vi "instrumentProperties_channel_gainLevels_init.vi"(8 "error in (no error)":errorcluster, 11 "OSAchannel in":refnum<class "OSAchannel.lvclass">) -> (0 "error out":errorcluster, 2 "gain values (relative)":dbl[](array[numeric]), 3 "OSAchannel out":refnum<class "OSAchannel.lvclass">)   [LabVIEW 2010, in "OSAchannel.lvclass"]
uses:
  OSAchannel.lvclass
  _dll/LVLib/FTSLib.lvlib
  OSA20X_misc.lvlib
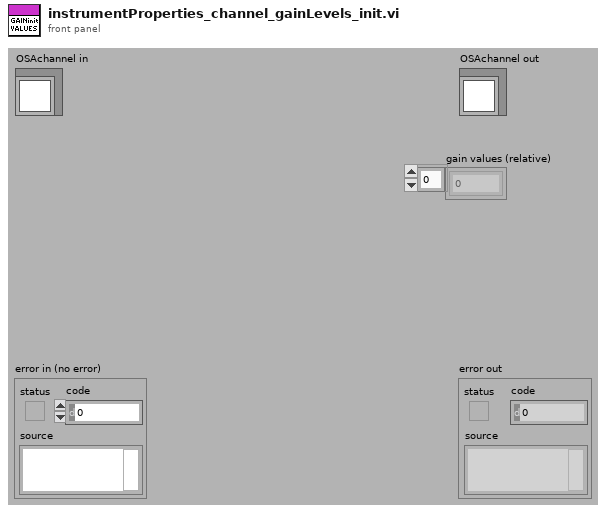
[diagram p1: front panel]
types:
  T1 = typedef "OSA20X_misc.lvlib/amplifier_sort.ctl" = enum16{"amp_unknown", "amp_se_8", "amp_se_12_lg", "amp_se_12", "amp_se_16", "amp_diff_8", "amp_diff_12_lg", "amp_diff_12_ir", "amp_diff_16", "amp_other", "amp_other_2"}
  T2 = typedef "OSA20X_misc.lvlib/detector_sort.ctl" = enum16{"unknown", "Silicon", "Silicon PIN", "Silicon MPPC", "InGaAs", "InGaAs ext low", "InGaAs ext high", "InAs", "InAsSb", "InSb", "MCT", "other", "other2", "other3"}
  T3 = typedef "OSA20X_misc.lvlib/interferogram_smoothing.ctl" = enum16{"NONE", "BINOMIAL", "SAVITSKY_GOLAY", "FOURIER", "MOVING_AVERAGE", "GAUSSIAN"}
  T4 = typedef "OSA20X_misc.lvlib/PDTemperatureMode.ctl" = enum16{"cool: better sensitivity/noise floor", "warm: extended wl range"}
  T5 = cluster{"waveMin (cm-1)":sgl, "waveMax (cm-1)":sgl, "gainOffset_auto":bool, "gain":i32, "gain levels nr":u16, "offset":i32, "offset max":u16, "damper available":bool, "damper active":bool, "amplifier sort":T1, "detector sort":T2, "channelIdx global":u16, "spectrIdx":u16, "waveMeter on":bool, "ref gainLevels rel.":refnum<data-value>, "intfgrm_smooth_width":u16, "intfgrm_smooth_nrOfPasses":u16, "intfgrm_smooth":T3, "adc #bits":u16, "temp Variable":bool, "spectr_smooth":T3, "spectr_smooth_width":u16, "spectr_smooth_nrOfPasses":u16, "PD sensitivity mode":T4, "damper auto":bool}
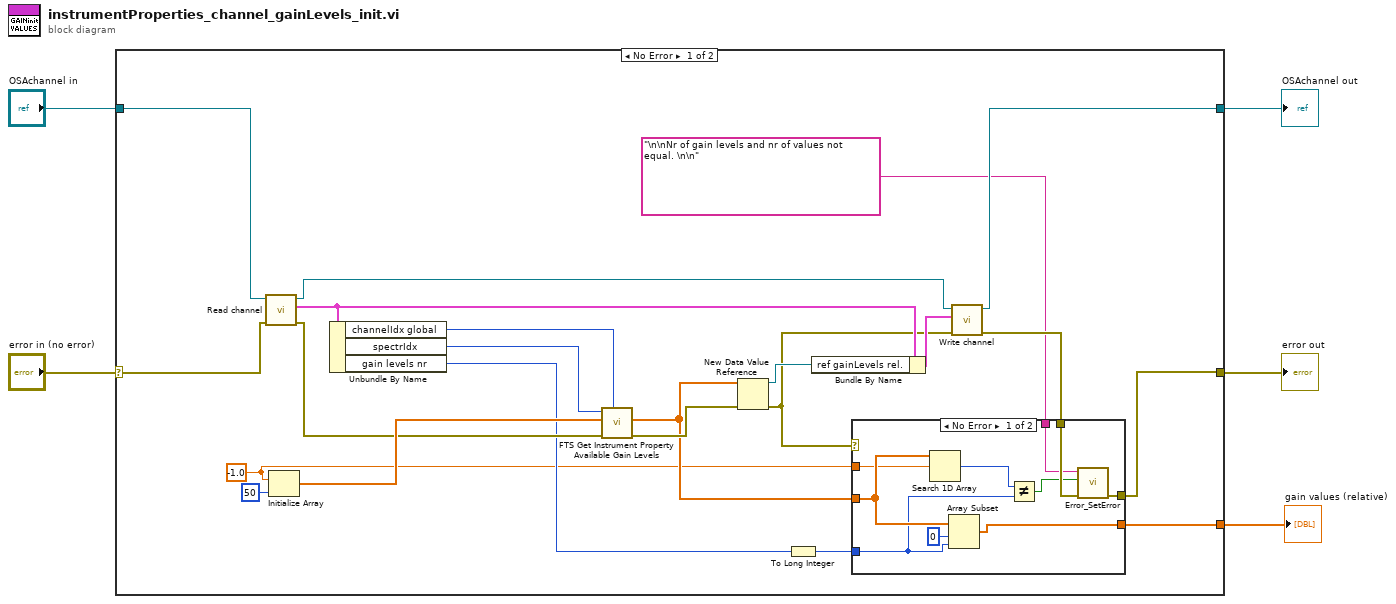
[diagram p0: block diagram]
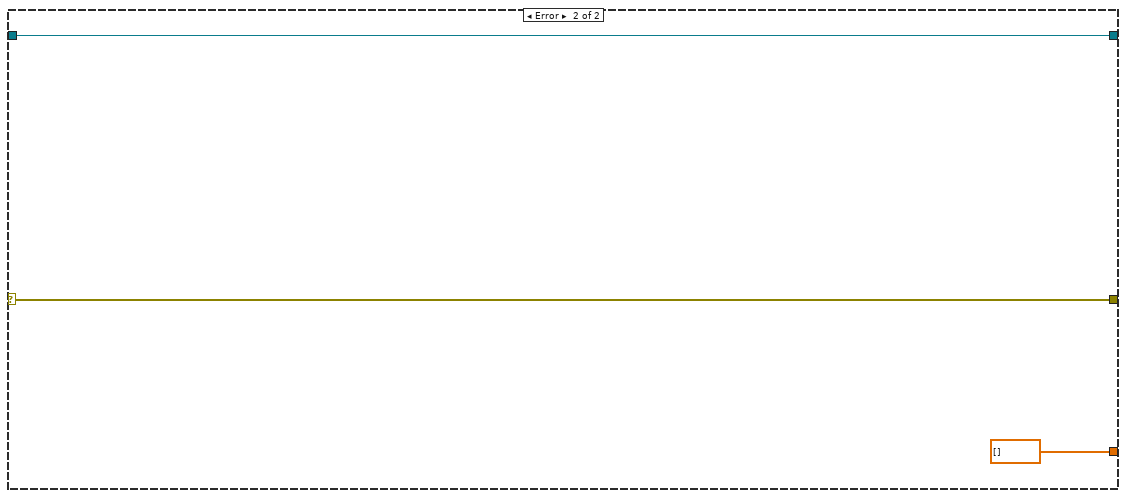
[diagram p3: hidden frame]
diagram:
  n1 = case shown="No Error" "error in (no error)" {
    selector: "error in (no error)" -> [w6 w42]
    tunnel: [w9 w42] -> w4
    tunnel: [w17 w41] -> w2
    tunnel: "OSAchannel in" -> [w18 w41]
    tunnel: [w8 dbl[] [] ("GainLevels out")] -> w1
    frame No Error {
      w13 = -1.0
      n2 = call "Read channel.vi"("error in (no error)"=w6, "OSAchannel in"=w18) -> ("error out"=w23:errorcluster, "channel"=w20:T5, "OSAchannel out"=w21:refnum<class "OSAchannel.lvclass">)  [unwired: 7 in]
      n3 = Initialize Array(w13, 50 ("dimension size")) -> (w24:dbl[])
      n4 = Unbundle By Name(w20) -> ("channelIdx global"=w25:u16, "spectrIdx"=w26:u16, "gain levels nr"=w15:u16)
      n5 = call "FTS Get Instrument Property Available Gain Levels.vi"("channel"=w25, "error in (no error)"=w23, "GainLevels"=w24, "specIndex"=w26) -> ("error out"=w22:errorcluster, "GainLevels out"=w14:dbl[])  [unwired: 5 in, 1 out]
      n6 = New Data Value Reference(data value=w14, error in=w22) -> (data value reference=w16:refnum<data-value>, error out=w7:errorcluster)
      n7 = To Long Integer(number=w15) -> (32bit integer=w12:i32)
      n8 = Bundle By Name(cluster=w20, "ref gainLevels rel."=w16) -> (w19:T5)
      n9 = call "Write channel.vi"("error in (no error)"=w7, "channel"=w19, "OSAchannel in"=w21) -> ("error out"=w11:errorcluster, "OSAchannel out"=w17:refnum<class "OSAchannel.lvclass">)  [unwired: 7 in]
      n10 = case shown="No Error" w7 {
        selector: w7 -> [_ w38]
        tunnel: w14 -> [w36 w39]
        tunnel: w13 -> [w35 _]
        tunnel: w12 -> [w34 _]
        tunnel: w11 -> [w33 _]
        tunnel: "\n\nNr of gain levels and nr of values not equal. \n\n" ("source(\"\")") -> [w32 _]
        tunnel: [w31 w38] -> w9
        tunnel: [w30 w39] -> w8
        frame No Error {
          n11 = Search 1D Array(1D array=w36, element=w35) -> (index of element=w29:i32)  [unwired: 1 in]
          n12 = Array Subset(array=w36, index=0, length=w34) -> (w30:dbl[])
          n13 = Not Equal?(x=w29, y=w34) -> (x != y?=w28:bool)
          n14 = call "Error_SetError.vi"("error in"=w33, "status (true)"=w28, "source(\"\")"=w32) -> ("error out"=w31:errorcluster)  [unwired: 4 in]
        }
        frame Error {
        }
      }
    }
    frame Error {
    }
  }
  "error out" <- w4
  "OSAchannel out" <- w2
  "gain values (relative)" <- w1
